vi "OperationCall.vi"(0 "Multiply in":refnum<class "Multiply.lvclass">, 5 "Sub Panel":refnum<vi>, 7 "user event out":refnum<user-event>, 9 "event source":refnum<user-event>, 11 "error in (no error)":errorcluster) -> (4 "Multiply out":refnum<class "Multiply.lvclass">, 15 "error out":errorcluster)   [LabVIEW 2023, in "Multiply.lvclass"]
uses:
  Multiply.lvclass
  Arithmetic/Arithmetic.lvclass
  MultiplicationUI.vi
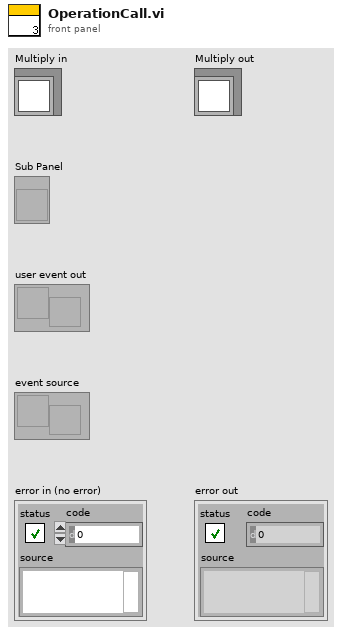
[diagram p1: front panel]
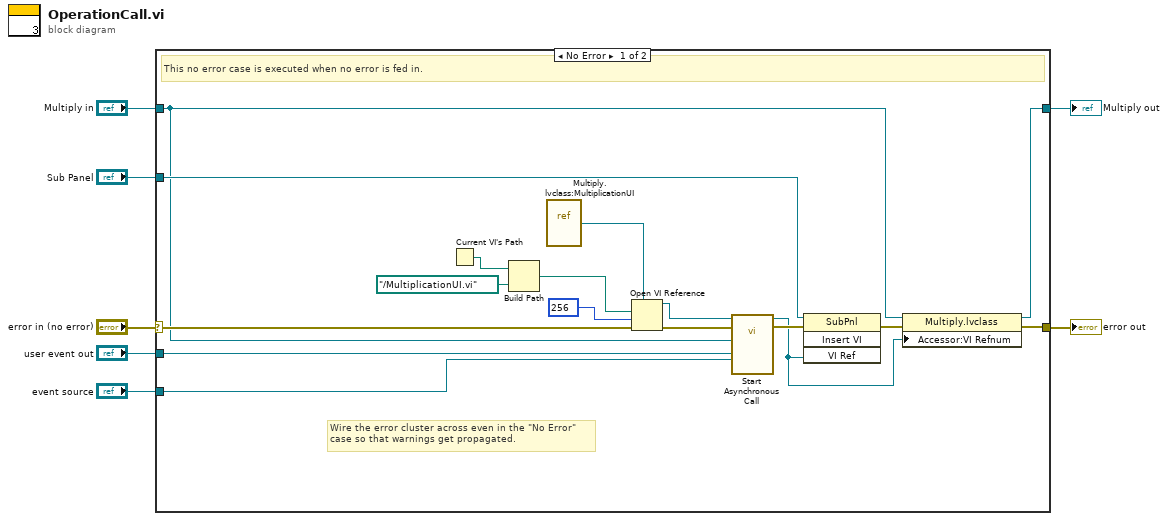
[diagram p0: block diagram]
diagram:
  n1 = case shown="No Error" "error in (no error)" {
    selector: "error in (no error)" -> [w19 w26]
    tunnel: [w14 w26] -> w6
    tunnel: [w13 w25] -> w4
    tunnel: "Multiply in" -> [w11 w25]
    tunnel: "user event out" -> [w17 _]
    tunnel: "event source" -> [w15 _]
    tunnel: "Sub Panel" -> [w16 _]
    frame No Error {
      # "Wire the error cluster across even in the \"No Error\"\ncase so that warnings get propagated."
      # "This no error case is executed when no error is fed in."
      n2 = Current VI's Path() -> (path=w9:path)
      n3 = Build Path(base path=w9, name or relative path=path "../MultiplicationUI.vi") -> (appended path=w8:path)
      n4 = vi-ref "Multiply.lvclass:MultiplicationUI.vi"() -> (w24:refnum<vi>)
      n5 = Open VI Reference(type specifier VI Refnum (for type only)=w24, vi path=w8, options=256, error in (no error)=w19) -> (vi reference=w20:refnum<vi>, error out=w22:errorcluster)  [unwired: 2 in]
      n6 = call-by-ref "Start Asynchronous Call"(reference=w20, error in=w22, "Multiply in"=w11, "user event out"=w17, "event source"=w15) -> (reference out=w12:refnum<vi>, error out=w23:errorcluster)  [unwired: 10 in, 3 out]
      n7 = invoke on="Invoke Node" class="SubPnl" method="Insert VI"(reference=w16, error in=w23, "VI Ref"=w12) -> (error out=w18:errorcluster)  [unwired: 1 in, 3 out]
      n8 = property class="Multiply.lvclass"(reference=w11, error in=w18, "Accessor:VI Refnum"=w12) -> (reference out=w13:refnum<class "Multiply.lvclass">, error out=w14:errorcluster)
    }
    frame Error {
      # "This error case is executed when error is fed in and fed out through error out."
    }
  }
  "error out" <- w6
  "Multiply out" <- w4
